vi "Set Enable State on Multiple Controls.vi"(8 "Error In":errorcluster, 10 "Disabled State":T1(ring), 11 "Controls":refnum<vi>[](array[refnum])) -> (0 "Error Out":errorcluster)   [LabVIEW 2015]
doc: "Sets all the controls in the input array to the \"Enable state\" value."
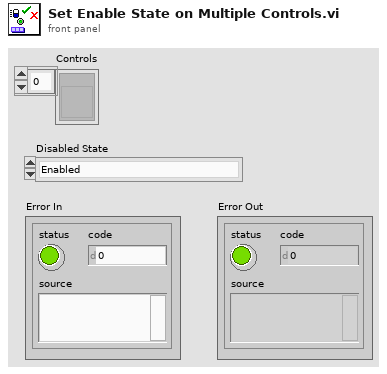
[diagram p1: front panel]
types:
  T1 = enum8{"Enabled", "Disabled", "Disabled and Grayed Out"}
  T2 = enum16{"None", "On Hover", "On Key Focus", "On Hover or Key Focus"}
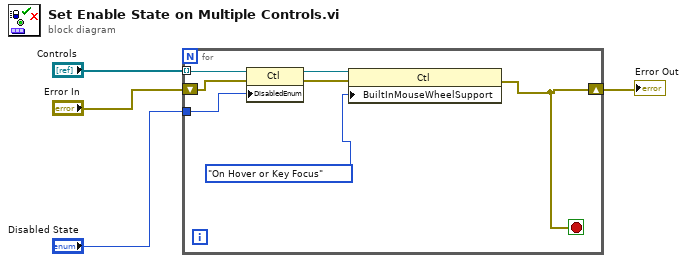
[diagram p0: block diagram]
diagram:
  n1 = for {
    tunnel: "Controls" -> [w11] mode=indexing
    tunnel: "Disabled State" -> [w10]
    shift-right: [w6] -> w3
    shift-left: "Error In" -> [w9]
    stop <- w6 stop-if-true
    n2 = property class="Ctl"(reference=w11, error in=w9, "DisabledEnum"=w10) -> (reference out=w8:refnum<vi>, error out=w7:errorcluster)
    n3 = property class="Ctl"(reference=w8, error in=w7, "BuiltInMouseWheelSupport"=T2."On Hover or Key Focus" ("Built-In Mouse Wheel Support")) -> (error out=w6:errorcluster)  [unwired: 1 out]
  }
  "Error Out" <- w3
